vi "acctoperbincounts.vi"(1 "accumulative counts":u32[](array[numeric])) -> (0 "counts per bin":u32[](array[numeric]))   [LabVIEW 2015]
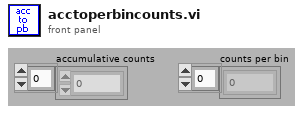
[diagram p1: front panel]
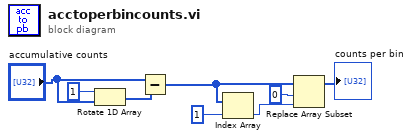
[diagram p0: block diagram]
diagram:
  n1 = Rotate 1D Array(1:"accumulative counts", 2:1 ("n")) -> (0:w2:u32[])
  n2 = Subtract(x="accumulative counts", y=w2) -> (x-y=w4:u32[])
  n3 = Index Array(array=w4, index=1) -> (element=w5:u32)
  n4 = Replace Array Subset(array=w4, new element=w5, index=0) -> (→"counts per bin":u32[])
